vi "Open_serial.vi"(4 "error in (no error)":errorcluster, 6 "Device serial (0=any)":u32 max=999999) -> (0 "error out":errorcluster, 3 "Device handle":u32 format="%x")   [LabVIEW 2014, in "MBUG-2820.lvlib"]
doc: "Opens a device specified by its serial number (last 6 digits of the id string). Pass 0 to open the firstavailable device.\nReturns a device handle which must be passed to all functions accessing the device."
uses:
  <instrlib>/MBUG-2820/MBUG-2820.lvlib
  <instrlib>/MBUG-2820/mbugdll.dll
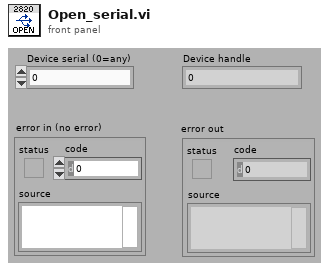
[diagram p1: front panel]
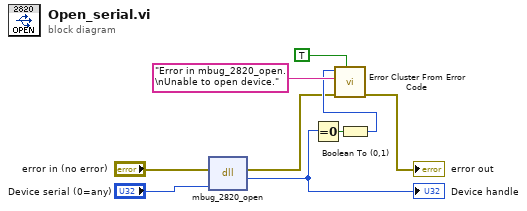
[diagram p0: block diagram]
diagram:
  n1 = dll-call lib="C:/Programme/National Instruments/LabVIEW 2014/instr.lib/MBUG-2820/mbugdll.dll" fn="mbug_2820_open"(error in="error in (no error)", "serial_num"="Device serial (0=any)") -> (error out=w2:errorcluster, "dev_handle"=w6:u64)  [unwired: 3 in, 1 out]
  "Device handle" <- w6
  n2 = Equal To 0?(x=w6) -> (x = 0?=w4:bool)
  n3 = Boolean To (0,1)(Boolean=w4) -> (0, 1=w3:i16)
  n4 = call <vilib>:"Error Cluster From Error Code.vi"("show call chain? (False)"=TRUE, "error in (no error)"=w2, "error message (\"\")"="Error in mbug_2820_open.\nUnable to open device.", "error code (0)"=w3) -> ("error out"=→"error out":errorcluster)  [unwired: 5 in]
